vi "Get image delay.vi"(8 "error in (no error)":errorcluster, 11 "CCDCamera in":refnum<class "Ixon_Ultra.lvclass">) -> (0 "error out":errorcluster, 3 "CCDCamera out":refnum<class "Ixon_Ultra.lvclass">)   [LabVIEW 2018, in "Ixon_Ultra.lvclass"]
doc: "Get the delay of the start of an exposure from the start of a kinetic series.\n\nThis function should only be used in a kinetic series with two or more frames."
uses:
  Ixon_Ultra.lvclass
  C:/Users/Denis/Desktop/S4ACS/S4ACS/Simulated_CCD_Camera/Simulated Camera.lvclass
  Simulated_CCD_Camera/Simulated Camera.lvclass
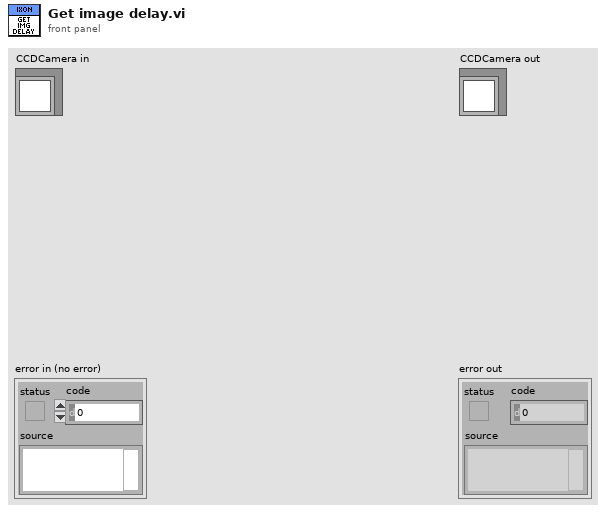
[diagram p1: front panel]
types:
  T1 = cluster{"FRAMES_DONE":u16, "CCD_STATUS":string, "CURRENT_TEMPERATURE":i16, "TEMPERATURE_STATUS":string, "FRAME_EXPOSURE_TIME":sgl, "SERIAL_NUMBER":u16, "ACQUIRING":bool, "POWER":bool}
  T2 = typedef "LVDateTimeRec.ctl" = cluster{"fractional second":dbl, "second":i32, "minute":i32, "hour":i32, "day of month":i32, "month":i32, "year":i32, "day of week":i32, "day of year":i32, "DST":i32}
  T3 = cluster{"Time Acq Started":u32, "Image delay":u64, "Last update - CCD config":timestamp, "SYSTEMTIME":T2, "Readout time":dbl, "Time acq finished":u32, "effective exptime":dbl}
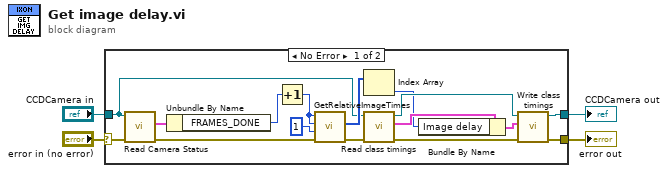
[diagram p0: block diagram]
diagram:
  n1 = case shown="No Error" "error in (no error)" {
    selector: "error in (no error)" -> [w18 w21]
    tunnel: "CCDCamera in" -> [w8 w22]
    tunnel: [w7 w22] -> w2
    tunnel: [w6 w21] -> w1
    frame No Error {
      n2 = call "Read Camera Status.vi"("error in (no error)"=w18, "CCDCamera in"=w8) -> ("error out"=w17:errorcluster, "camera status"=w16:T1)  [unwired: 7 in, 1 out]
      n3 = Unbundle By Name(w16) -> ("FRAMES_DONE"=w15:u16)
      n4 = Increment(x=w15) -> (x+1=w14:u16)
      n5 = call <userlib>:"GetRelativeImageTimes.vi"("error in (no error)"=w17, "size"=u32 1 ("first"), "last"=w14, "first"=w14) -> ("error out"=w9:errorcluster, "arr"=w19:u64[])  [unwired: 5 in, 1 out]
      n6 = Index Array(array=w19) -> (element=w5:u64)  [unwired: 1 in]
      n7 = call-dynamic "Read class timings.vi"("error in (no error)"=w9, "Simulated Camera in"=w8) -> ("error out"=w11:errorcluster, "class timings"=w10:T3, "Simulated Camera out"=w12:refnum<class "Ixon_Ultra.lvclass">)  [unwired: 7 in]
      n8 = Bundle By Name(cluster=w10, "Image delay"=w5) -> (w13:T3)
      n9 = call-dynamic "Write class timings.vi"("error in (no error)"=w11, "class timings"=w13, "Simulated Camera in"=w12) -> ("error out"=w6:errorcluster, "Simulated Camera out"=w7:refnum<class "Ixon_Ultra.lvclass">)  [unwired: 7 in]
    }
    frame Error {
    }
  }
  "error out" <- w1
  "CCDCamera out" <- w2
